vi "Get QDAcroynm and QD File Path Base on QDFullname.vi"(8 "error in (no error)":errorcluster, 10 "QDFunctions(\"\")":string, 11 "QDDialogList in":refnum<class "QDDialogList.lvclass">) -> (0 "error out":errorcluster, 1 "QD File Path(\"\")":string, 2 "QD Acronym(\"\")":string, 3 "QDDialogList out":refnum<class "QDDialogList.lvclass">)   [LabVIEW 2015, in "QDDialogList.lvclass"]
uses:
  QDDialogList.lvclass
  QDDialogList.lvclass/QDDialogList.ctl
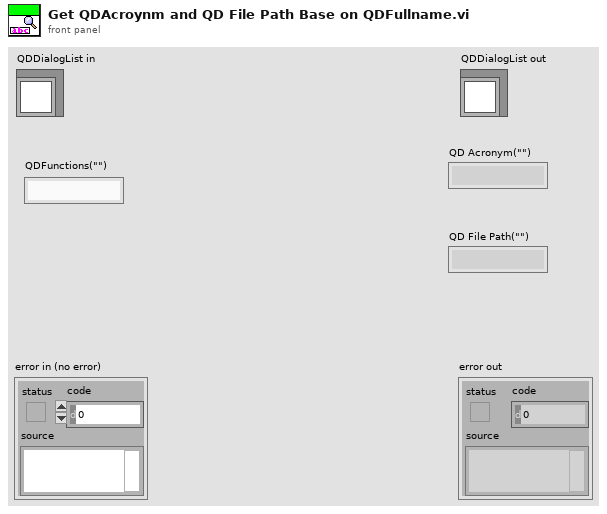
[diagram p1: front panel]
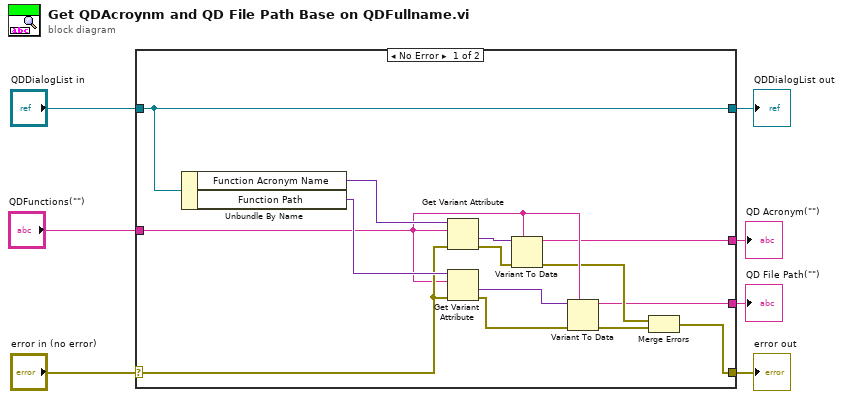
[diagram p0: block diagram]
diagram:
  n1 = case shown="No Error" "error in (no error)" {
    selector: "error in (no error)" -> [w18 w23]
    tunnel: [w10 w23] -> w6
    tunnel: [w21 w22] -> w4
    tunnel: "QDDialogList in" -> [w21 w22]
    tunnel: "QDFunctions(\"\")" -> [w13 _]
    tunnel: [w9 _] -> w2
    tunnel: [w8 _] -> w1
    frame No Error {
      n2 = Unbundle By Name(w21) -> ("Function Acronym Name"=w20:variant, "Function Path"=w19:variant)
      n3 = Get Variant Attribute(Variant=w20, name=w13, error in=w18) -> (value=w17:variant, error out=w16:errorcluster)  [unwired: 1 in, 2 out]
      n4 = Get Variant Attribute(Variant=w19, name=w13, error in=w18) -> (value=w14:variant, error out=w15:errorcluster)  [unwired: 1 in, 2 out]
      n5 = Variant To Data(error in=w16, type=w13, Variant=w17) -> (data=w9:string, error out=w11:errorcluster)
      n6 = Variant To Data(error in=w15, type=w13, Variant=w14) -> (data=w8:string, error out=w12:errorcluster)
      n7 = Merge Errors(w11, w12) -> (w10:errorcluster)
    }
    frame Error {
    }
  }
  "error out" <- w6
  "QDDialogList out" <- w4
  "QD Acronym(\"\")" <- w2
  "QD File Path(\"\")" <- w1
